vi "Read.vi"(0 "Path":path, 11 "error in (no error)":errorcluster) -> (4 "FSM.Graph":refnum<class "FSM.Graph.lvclass">, 10 "Success":bool, 15 "error out":errorcluster)   [LabVIEW 2020, in "FSM.Graph.lvclass"]
uses:
  FSM.Graph.lvclass
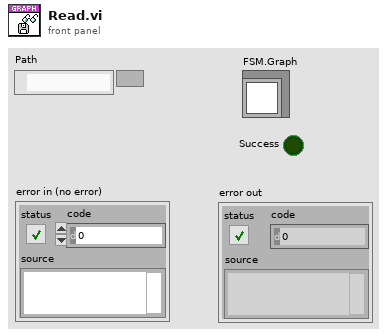
[diagram p1: front panel]
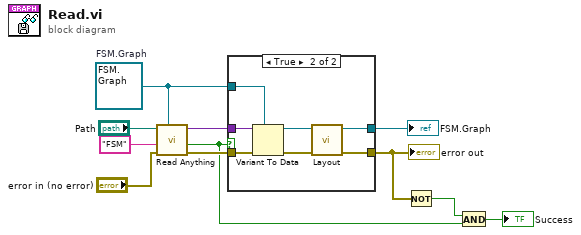
[diagram p0: block diagram]
diagram:
  w8 = refnum<class "FSM.Graph.lvclass"> refnum  # FSM.Graph
  n1 = call "Read Anything.vi"("Type of Anything"=w8, "Error In"="error in (no error)", "Section Name (Name of \"Type of Anything\")"="FSM" ("Section Name (Name of \"Type of Anything\")"), "Path (dialog)"="Path") -> ("Error Out"=w10:errorcluster, "Found?"=w4:bool, "Anything"=w9:variant)  [unwired: 5 in]
  n2 = case shown="True" w4 {
    tunnel: w10 -> [w12 w19]
    tunnel: w9 -> [_ w18]
    tunnel: w8 -> [_ w17]
    tunnel: [_ w14] -> w5
    tunnel: [w12 w13] -> w2
    frame False {
    }
    frame True {
      n3 = Variant To Data(error in=w19, type=w17, Variant=w18) -> (data=w15:refnum<class "FSM.Graph.lvclass">, error out=w16:errorcluster)
      n4 = call "Layout.vi"("error in (no error)"=w16, "FSM in"=w15) -> ("error out"=w13:errorcluster, "FSM out"=w14:refnum<class "FSM.Graph.lvclass">)  [unwired: 8 in]
    }
  }
  "error out" <- w2
  "FSM.Graph" <- w5
  n5 = Not(x=w2) -> (.not. x?=w3:bool)
  n6 = And(x=w3, y=w4) -> (x .and. y?=→"Success":bool)
